vi "test PHD2000 pump.vi"() -> ()   [LabVIEW 2017]
uses:
  <instrlib>/Harvard Syringe Pump PHD2000/Harvard Syringe Pump PHD2000.lvlib
panel:
  out "error out":errorcluster
  in  "Boolean":bool
  in  "Target (ml)":dbl min=0.0 max=50.0 format="%#.3g"
  out "Pump stop":bool
  in  "VISA resource name":refnum<visa-resource-name>
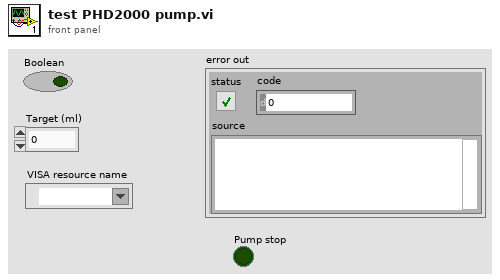
[diagram p1: front panel]
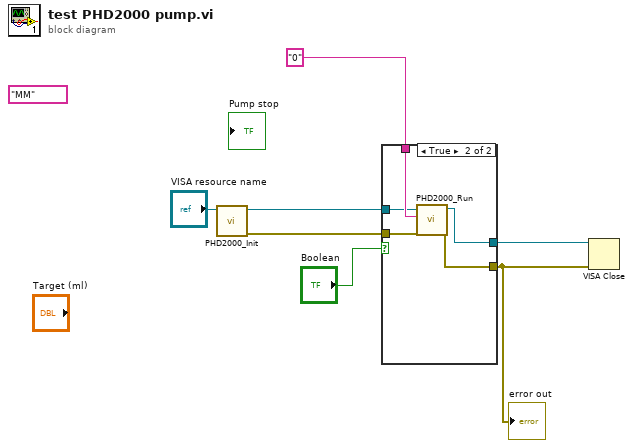
[diagram p0: block diagram]
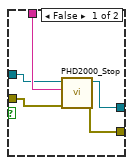
[diagram p2: hidden frame]
diagram:
  (unwired) "MM" ("Unit")
  n1 = call <instrlib>:"PHD2000_Init.vi"("VISA resource name"="VISA resource name") -> ("error out"=w2:errorcluster, "reference out"=w3:refnum<visa-resource-name>)  [unwired: 8 in]
  n2 = case shown="True" "Boolean" {
    tunnel: [w12 w17] -> w5
    tunnel: [w11 w16] -> w1
    tunnel: "0" ("Pump #") -> [w10 w15]
    tunnel: w3 -> [w9 w14]
    tunnel: w2 -> [w8 w13]
    frame False {
      n3 = call <instrlib>:"PHD2000_Stop.vi"("VISA resource name 2"=w9, "Pump #"=w10, "error in (no error)"=w8) -> ("VISA resource name out"=w12:refnum<visa-resource-name>, "error out"=w11:errorcluster)  [unwired: 6 in]
    }
    frame True {
      n4 = call <instrlib>:"PHD2000_Run.vi"("VISA resource name 2"=w14, "Pump #"=w15, "error in (no error)"=w13) -> ("VISA resource name out"=w17:refnum<visa-resource-name>, "error out"=w16:errorcluster)  [unwired: 6 in]
    }
  }
  "error out" <- w1
  n5 = VISA Close(VISA resource name=w5, error in (no error)=w1) -> ()  [unwired: 1 out]
